vi "FSK_RFLoopback1.vi"(5 "xsrpip":string, 7 "pcip":string, 8 "error in (no error)":errorcluster caption="错误输入（无错误）", 10 "SendSig":dbl[](array[numeric]), 11 "PathIn":path) -> (0 "error out":errorcluster caption="错误输出", 2 "RecvSig":dbl[](array[numeric]), 3 "PathOut":path)   [LabVIEW 2015]
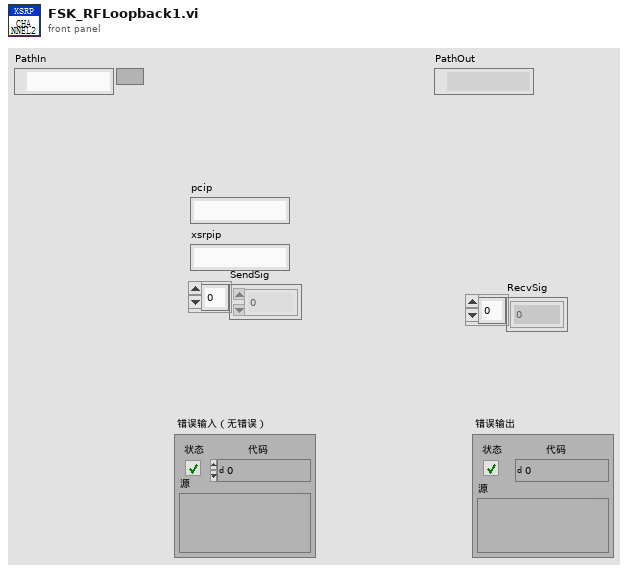
[diagram p1: front panel]
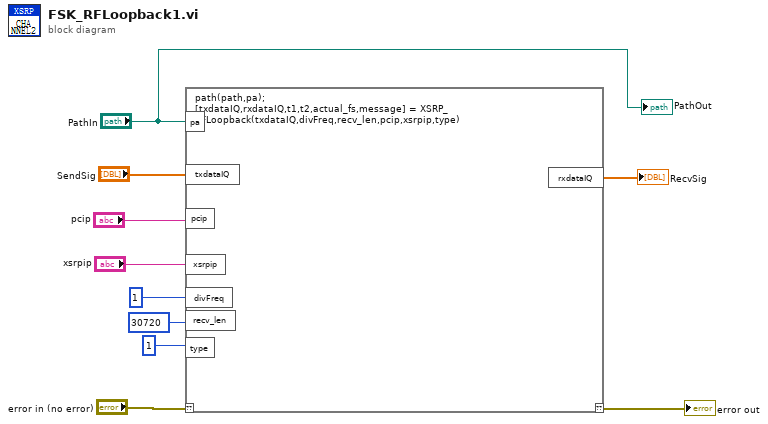
[diagram p0: block diagram]
diagram:
  n1 = script code="path(path,pa);\n[txdataIQ,rxdataIQ,t1,t2,actual_fs,message] = XSRP_RFLoopback(txdataIQ,divFreq,recv_len,pcip,xsrpip,type)"("??"="error in (no error)", "pa"="PathIn", "txdataIQ"="SendSig", "xsrpip"="xsrpip", "pcip"="pcip", "divFreq"=1, "recv_len"=30720, "type"=1) -> ("??"=→"error out":errorcluster, "rxdataIQ"=→"RecvSig":cdb[])
  "PathOut" <- "PathIn"
